vi "DQtoABC_noSine_UnitaryMagnitude_src.vi"(0 "d":sgl, 1 "cos":sgl, 2 "sin":sgl, 5 "q":sgl) -> (4 "a":sgl, 6 "b":sgl, 8 "c":sgl, 10 "alpha":sgl, 15 "beta":sgl)   [LabVIEW 2015]
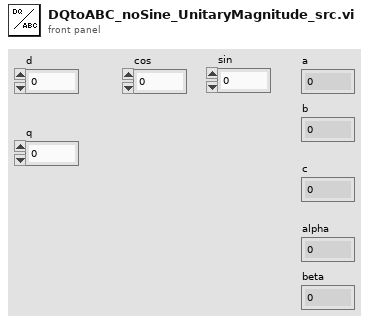
[diagram p1: front panel]
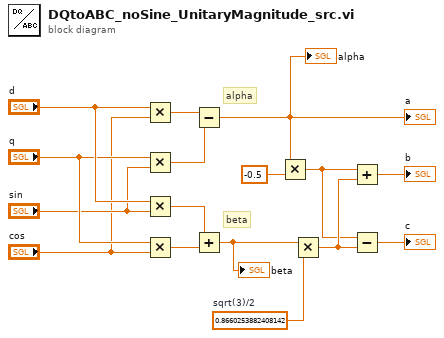
[diagram p0: block diagram]
diagram:
  w7 = sgl 0.8660254  # sqrt(3)/2
  # "beta"
  # "alpha"
  n1 = Multiply(x="d", y="cos") -> (x*y=w14:sgl)
  n2 = Multiply(x="q", y="sin") -> (x*y=w13:sgl)
  n3 = Multiply(x="d", y="sin") -> (x*y=w16:sgl)
  n4 = Multiply(x="q", y="cos") -> (x*y=w15:sgl)
  n5 = Subtract(x=w14, y=w13) -> (x-y=w10:sgl)
  "a" <- w10
  "alpha" <- w10
  n6 = Add(x=w16, y=w15) -> (x+y=w8:sgl)
  "beta" <- w8
  n7 = Multiply(x=w10, y=sgl -0.5) -> (x*y=w4:sgl)
  n8 = Multiply(x=w8, y=w7) -> (x*y=w5:sgl)
  n9 = Add(x=w4, y=w5) -> (x+y=→"b":sgl)
  n10 = Subtract(x=w4, y=w5) -> (x-y=→"c":sgl)
